vi "Staage 3.vi"() -> (0 "pass":bool=TRUE, 1 "Boolean 5":bool, 2 "Boolean 7":bool, 3 "Boolean 8":bool)   [LabVIEW 2014]
uses:
  <vilib>/Utility/miscctls.llb/LVPositionTypeDef.ctl
panel:
  in  "Position 2":T1={"Left"=24, "Top"=2148}
  in  "hh":dbl format="%0#2_6g"
  in  ":":dbl format="%0#2_6g"
  in  "ss":dbl format="%0#2_6g"
  in  "OK Button 112":bool
  out "Boolean 3":bool
  out "Boolean":bool
  out "Boolean 2":bool
  out "star 1":bool
  out "star 2":bool
  out "star 3":bool
  out "result":bool
  in  "Boolean 6":bool
  in  "Position":T1
  in  "Map Array":dbl[][](array[numeric])=array190x190[36100 elements]
  in  "OK Button 111":bool
  in  "OK Button 110":bool
  in  "OK Button 109":bool
  in  "OK Button 108":bool
  in  "OK Button 107":bool
  in  "OK Button 106":bool
  in  "OK Button 105":bool
  in  "OK Button 104":bool
  in  "OK Button 103":bool
  in  "OK Button 102":bool
  in  "OK Button 101":bool
  in  "OK Button 100":bool
  in  "OK Button 99":bool
  in  "OK Button 98":bool
  in  "OK Button 97":bool
  in  "OK Button 96":bool
  in  "OK Button 95":bool
  in  "OK Button 94":bool
  in  "stop 4":bool
  in  "OK Button 93":bool
  in  "OK Button 92":bool
  in  "OK Button 91":bool
  in  "OK Button 90":bool
  in  "OK Button 89":bool
  in  "OK Button 88":bool
  in  "OK Button 87":bool
  in  "OK Button 86":bool
  in  "OK Button 85":bool
  in  "OK Button 84":bool
  in  "OK Button 83":bool
  in  "OK Button 82":bool
  in  "OK Button 81":bool
  in  "OK Button 80":bool
  in  "OK Button 79":bool
  in  "OK Button 78":bool
  in  "OK Button 77":bool
  in  "OK Button 76":bool
  in  "OK Button 75":bool
  in  "OK Button 74":bool
  in  "OK Button 73":bool
  in  "stop 3":bool
  in  "stop 2":bool
  in  "OK Button 72":bool
  in  "OK Button 71":bool
  in  "OK Button 70":bool
  in  "OK Button 69":bool
  in  "OK Button 68":bool
  in  "OK Button 67":bool
  in  "OK Button 66":bool
  in  "OK Button 65":bool
  in  "OK Button 64":bool
  in  "OK Button 63":bool
  in  "OK Button 62":bool
  in  "OK Button 61":bool
  in  "OK Button 60":bool
  in  "OK Button 59":bool
  in  "OK Button 58":bool
  in  "OK Button 57":bool
  in  "OK Button 56":bool
  in  "OK Button 55":bool
  in  "OK Button 54":bool
  in  "OK Button 53":bool
  in  "OK Button 52":bool
  in  "OK Button 51":bool
  in  "OK Button 50":bool
  in  "OK Button 49":bool
  in  "OK Button 48":bool
  in  "OK Button 47":bool
  in  "OK Button 46":bool
  in  "OK Button 45":bool
  in  "OK Button 44":bool
  in  "OK Button 43":bool
  in  "OK Button 42":bool
  in  "OK Button 41":bool
  in  "OK Button 40":bool
  in  "OK Button 39":bool
  in  "OK Button 38":bool
  in  "OK Button 37":bool
  in  "OK Button 36":bool
  in  "OK Button 35":bool
  in  "OK Button 34":bool
  in  "OK Button 33":bool
  in  "OK Button 32":bool
  in  "OK Button 31":bool
  in  "OK Button 30":bool
  in  "OK Button 29":bool
  in  "OK Button 28":bool
  in  "OK Button 27":bool
  in  "OK Button 26":bool
  in  "OK Button 25":bool
  in  "OK Button 24":bool
  in  "OK Button 23":bool
  in  "OK Button 22":bool
  in  "OK Button 21":bool
  in  "OK Button 20":bool
  in  "OK Button 19":bool
  in  "OK Button 18":bool
  in  "OK Button 17":bool
  in  "OK Button 16":bool
  in  "OK Button 15":bool
  in  "OK Button 14":bool
  in  "OK Button 13":bool
  in  "OK Button 12":bool
  in  "OK Button 11":bool
  in  "OK Button 10":bool
  in  "OK Button 9":bool
  in  "OK Button 8":bool
  in  "OK Button 7":bool
  in  "OK Button 6":bool
  in  "OK Button 5":bool
  in  "OK Button 4":bool
  in  "OK Button 3":bool
  in  "OK Button 2":bool
  in  "character":bool
  in  "OK Button":bool
  out "Boolean 4":bool
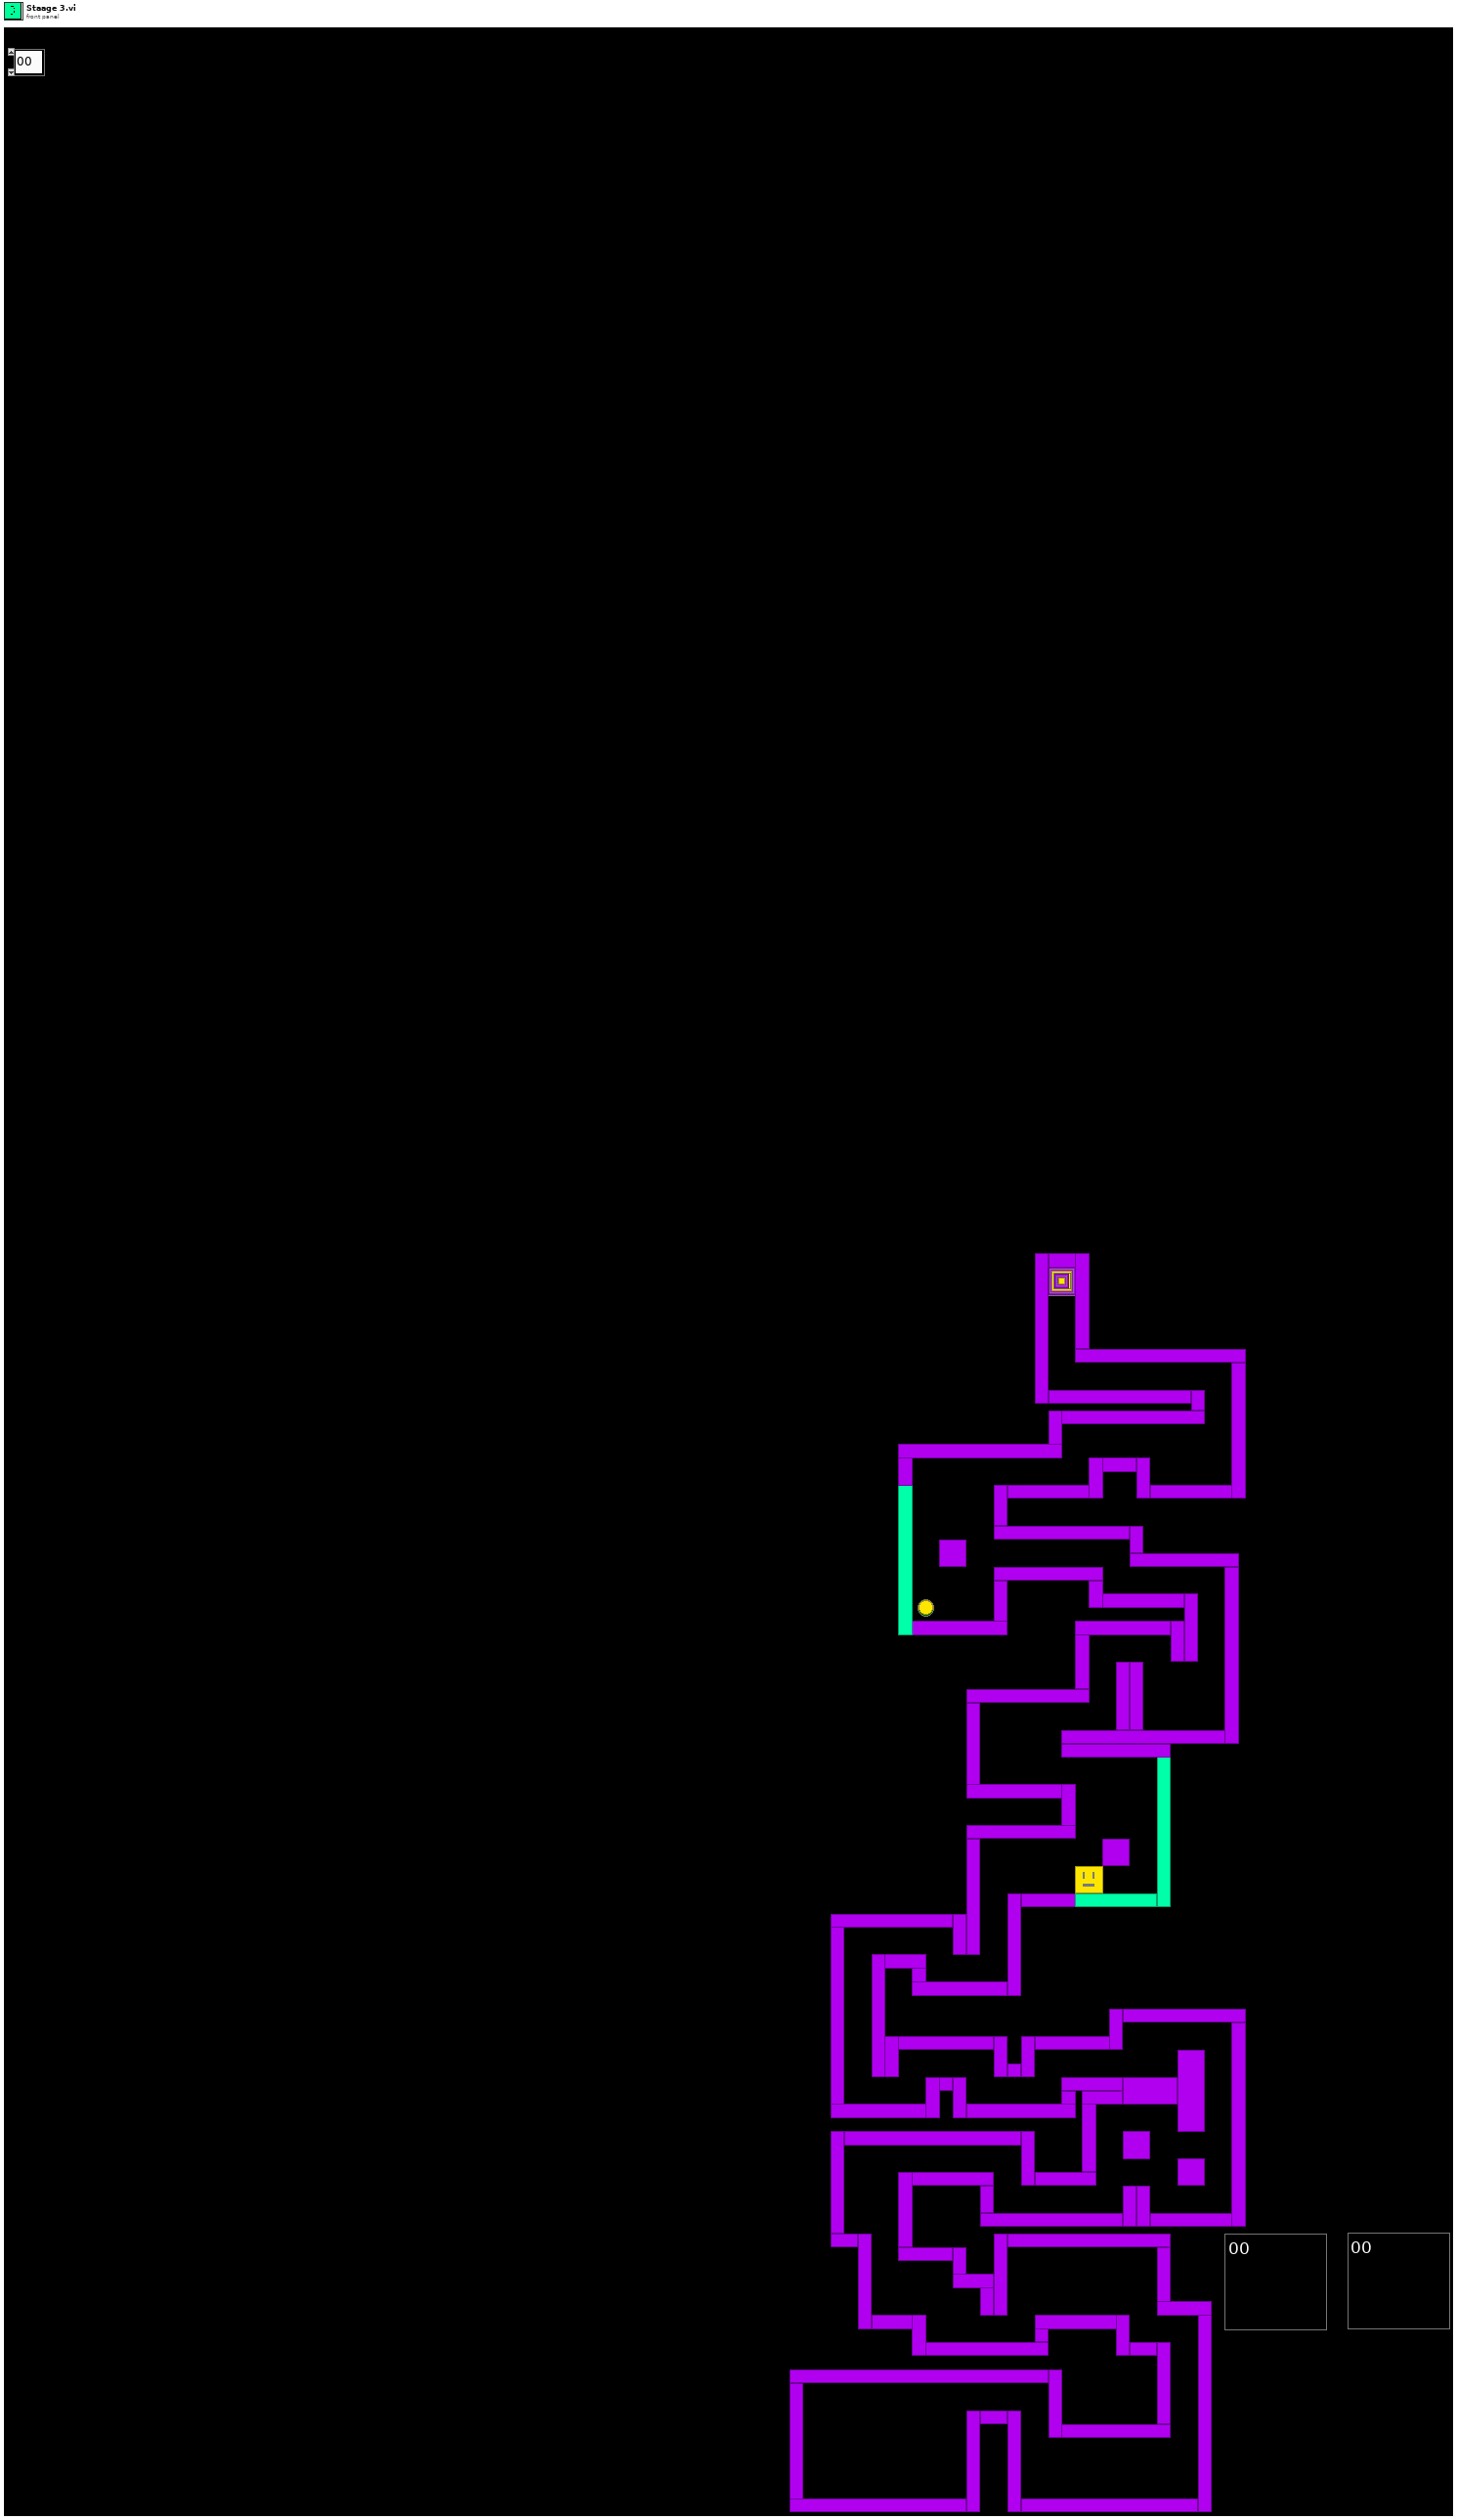
[diagram p1: front panel]
types:
  T1 = typedef "LVPositionTypeDef.ctl" = cluster{"Left":i32, "Top":i32}
  T2 = typedef "eventvkey.ctl" = enum16{"ASCII", "Enter", "Return", "Shift", "Ctrl", "Alt", "Cmd", "Opt", "Caps", "NumLock", "Clear", "Break", "Up", "Down", "Left", "Right", "Insert", "Delete", "Home", "End", "PageUp", "PageDown", "Escape", "Help", "Pause", "ScrollLock", "F1", "F2", "F3", "F4", "F5", "F6", "F7", "F8", "F9", "F10", "F11", "F12", "F13", "F14", "F15", "F16", "F17", "F18", "F19", "F20", "F21", "F22", "F23", "F24", "Play", "VolumeUp", "VolumeDown", "Mute", "Two Byte Char"}
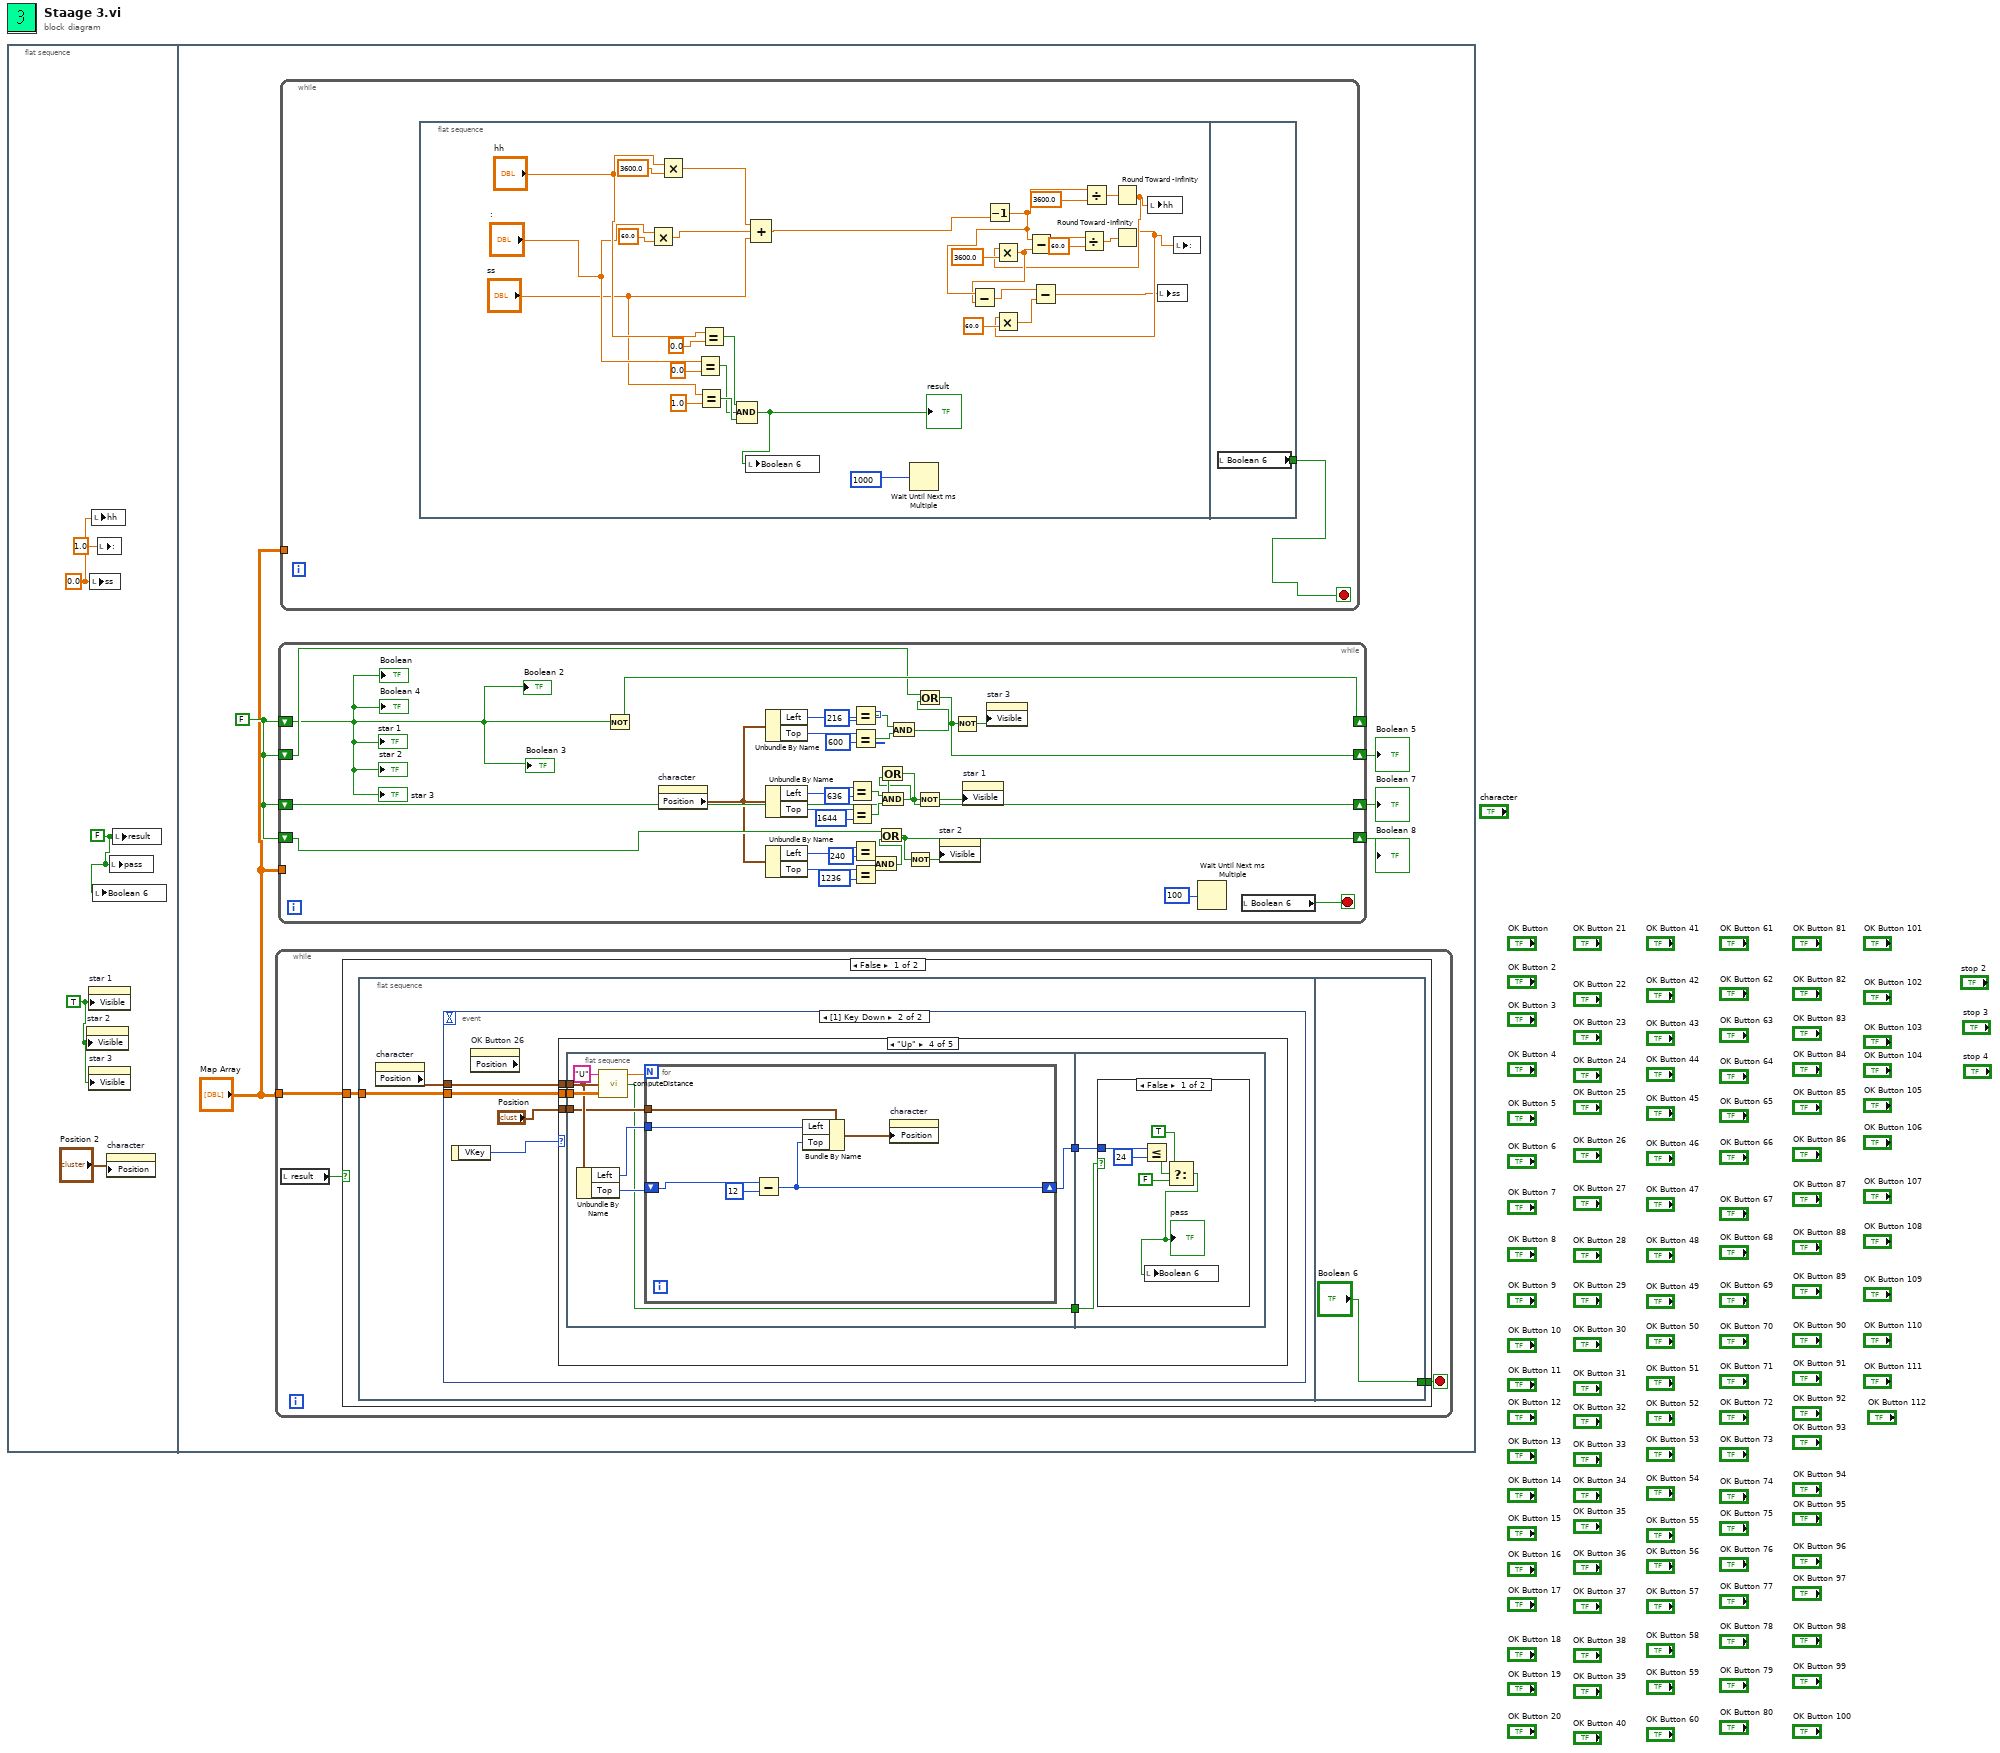
[diagram p0: block diagram]
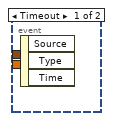
[diagram p2: hidden frame]
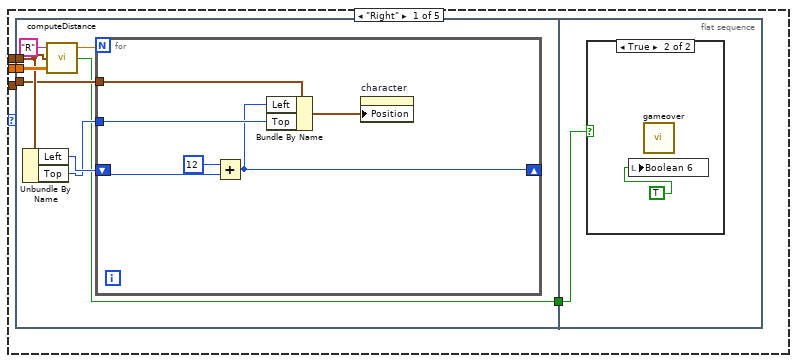
[diagram p3: hidden frame]
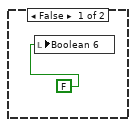
[diagram p4: hidden frame]
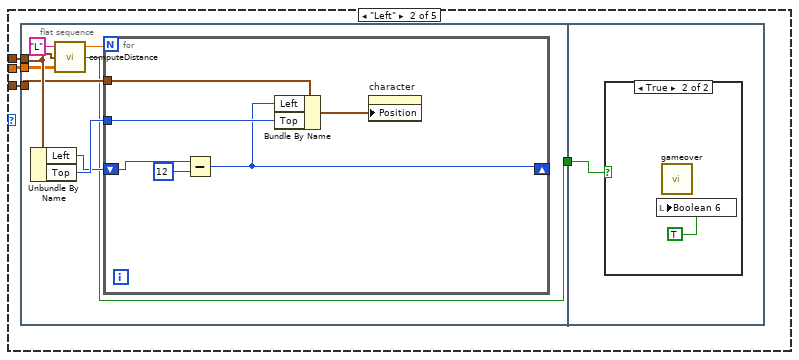
[diagram p5: hidden frame]
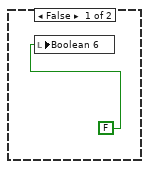
[diagram p6: hidden frame]
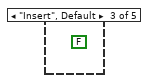
[diagram p7: hidden frame]
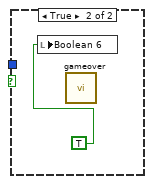
[diagram p8: hidden frame]
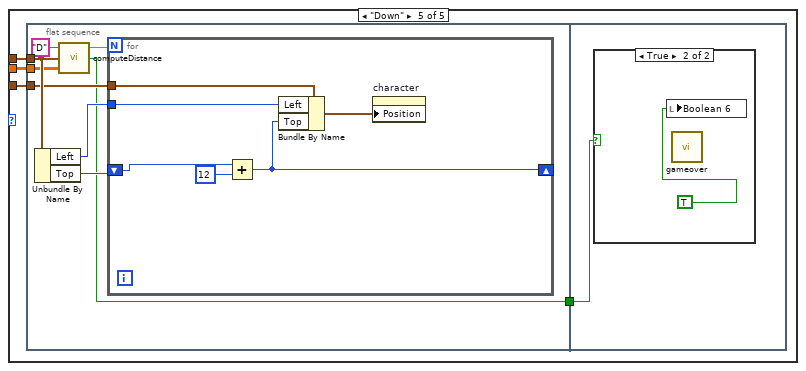
[diagram p9: hidden frame]
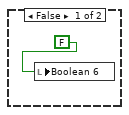
[diagram p10: hidden frame]
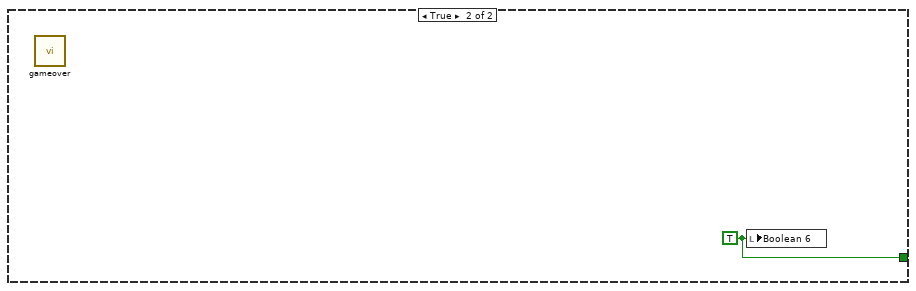
[diagram p11: hidden frame]
diagram:
  n1 = flat-sequence {
    frame #0 {
      w2 = TRUE ("Visible")
      w3 = FALSE ("result")
      w5 = 0.0 ("ss")
      n2 = property on="star 2" class="Bool (strict)"("Visible"=w2) -> ()  [unwired: 2 in, 2 out]
      n3 = property on="star 1" class="Bool (strict)"("Visible"=w2) -> ()  [unwired: 2 in, 2 out]
      n4 = property on="star 3" class="Bool (strict)"("Visible"=w2) -> ()  [unwired: 2 in, 2 out]
      n5 = local write "ss"(w5) -> ()
      n6 = local write "hh"(w5) -> ()
      n7 = local write "Boolean 6"(w3) -> ()
      n8 = local write ":"(1.0 (":")) -> ()
      n9 = property on="character" class="Bool"("Position"="Position 2") -> ()  [unwired: 2 in, 2 out]
      n10 = local write "pass"(w3) -> ()
      n11 = local write "result"(w3) -> ()
    }
    frame #1 {
      w10 = FALSE
      n12 = while {
        tunnel: "Map Array" -> [w80]
        stop <- w79 stop-if-true
        n13 = local read "result"() -> (w78:bool)
        n14 = case shown="False" w78 {
          tunnel: w80 -> [w82 _]
          tunnel: [w81 w182] -> w79
          frame False {
            n15 = flat-sequence {
              tunnel: w82 -> [w84]
              tunnel: ["Boolean 6"] -> w81
              frame #0 {
                n16 = property on="character" class="Bool"() -> ("Position"=w83:T1)  [unwired: 2 in, 2 out]
                n17 = event shown="[1] Key Down" {
                  selector: _ -> [_ _]
                  dyn-events: _ -> [_ _]
                  timeout: _ -> [_ _]
                  tunnel: w84 -> [_ w87]
                  tunnel: w83 -> [_ w86]
                  event Timeout {
                    n18 = event-data() -> ()  [unwired: 1 in, 3 out]
                  }
                  event Key Down {
                    n19 = event-data() -> ("VKey"=w88:T2)  [unwired: 1 in]
                    n20 = property on="OK Button 26" class="Bool" props=["Position"]() -> ()  [unwired: 2 in, 3 out]
                    n21 = case shown="\"Up\"" w88 {
                      tunnel: w87 -> [w92 w112 _ w135 w162]
                      tunnel: w86 -> [w91 w113 _ w134 w163]
                      tunnel: "Position" -> [w90 w111 _ w133 w161]
                      frame "Right" {
                        n22 = flat-sequence {
                          tunnel: w92 -> [w98]
                          tunnel: w91 -> [w97]
                          tunnel: w90 -> [w96]
                          tunnel: [w93] -> w89
                          tunnel: w89 -> [w107]
                          frame #0 {
                            n23 = Unbundle By Name(w97) -> ("Left"=w95:i32, "Top"=w94:i32)
                            n24 = call "computeDistance.vi"("Array"=w98, "Position"=w97, "String"="R") -> ("2"=w93:bool, "distance"=w100:dbl)  [unwired: 1 out]
                            n25 = for {
                              N: w100 -> [_]
                              shift-right: [w103] -> _
                              shift-left: w95 -> [w106]
                              tunnel: w96 -> [w105]
                              tunnel: w94 -> [w104]
                              n26 = Add(x=12, y=w106) -> (x+y=w103:i32)
                              n27 = Bundle By Name(cluster=w105, "Left"=w103, "Top"=w104) -> (w101:T1)
                              n28 = property on="character" class="Bool"("Position"=w101) -> ()  [unwired: 2 in, 2 out]
                            }
                          }
                          frame #1 {
                            n29 = case shown="True" w107 {
                              frame False {
                                n30 = local write "Boolean 6"(FALSE) -> ()
                              }
                              frame True {
                                n31 = local write "Boolean 6"(TRUE) -> ()
                                n32 = call "gameover.vi"() -> ()  [unwired: 1 in]
                              }
                            }
                          }
                        }
                      }
                      frame "Left" {
                        n33 = flat-sequence {
                          tunnel: w113 -> [w117]
                          tunnel: w112 -> [w116]
                          tunnel: w111 -> [w115]
                          tunnel: [w114] -> w110
                          tunnel: w110 -> [w128]
                          frame #0 {
                            n34 = Unbundle By Name(w117) -> ("Left"=w120:i32, "Top"=w121:i32)
                            n35 = call "computeDistance.vi"("Array"=w116, "Position"=w117, "String"="L") -> ("2"=w114:bool, "distance"=w118:dbl)  [unwired: 1 out]
                            n36 = for {
                              N: w118 -> [_]
                              shift-right: [w125] -> _
                              shift-left: w120 -> [w124]
                              tunnel: w115 -> [w127]
                              tunnel: w121 -> [w126]
                              n37 = Subtract(x=w124, y=12) -> (x-y=w125:i32)
                              n38 = Bundle By Name(cluster=w127, "Left"=w125, "Top"=w126) -> (w122:T1)
                              n39 = property on="character" class="Bool"("Position"=w122) -> ()  [unwired: 2 in, 2 out]
                            }
                          }
                          frame #1 {
                            n40 = case shown="True" w128 {
                              frame False {
                                n41 = local write "Boolean 6"(FALSE) -> ()
                              }
                              frame True {
                                n42 = local write "Boolean 6"(TRUE) -> ()
                                n43 = call "gameover.vi"() -> ()  [unwired: 1 in]
                              }
                            }
                          }
                        }
                      }
                      frame "Insert", Default {
                        (unwired) FALSE
                      }
                      frame "Up" {
                        n44 = flat-sequence {
                          tunnel: w135 -> [w144]
                          tunnel: w134 -> [w141]
                          tunnel: w133 -> [w138]
                          tunnel: [w137] -> w132
                          tunnel: [w136] -> w131
                          tunnel: w132 -> [w152]
                          tunnel: w131 -> [w151]
                          frame #0 {
                            n45 = Unbundle By Name(w141) -> ("Left"=w139:i32, "Top"=w140:i32)
                            n46 = call "computeDistance.vi"("Array"=w144, "Position"=w141, "String"="U") -> ("2"=w137:bool, "distance"=w142:dbl)  [unwired: 1 out]
                            n47 = for {
                              N: w142 -> [_]
                              shift-right: [w150] -> w136
                              shift-left: w140 -> [w147]
                              tunnel: w139 -> [w149]
                              tunnel: w138 -> [w148]
                              n48 = Subtract(x=w147, y=12) -> (x-y=w150:i32)
                              n49 = Bundle By Name(cluster=w148, "Left"=w149, "Top"=w150) -> (w145:T1)
                              n50 = property on="character" class="Bool"("Position"=w145) -> ()  [unwired: 2 in, 2 out]
                            }
                          }
                          frame #1 {
                            n51 = case shown="False" w152 {
                              tunnel: w151 -> [w158 _]
                              frame False {
                                n52 = Less Or Equal?(x=w158, y=24) -> (x <= y?=w156:bool)
                                n53 = Select(t=TRUE, s=w156, f=FALSE) -> (s? t:f=w154:bool)
                                "pass" <- w154
                                n54 = local write "Boolean 6"(w154) -> ()
                              }
                              frame True {
                                n55 = local write "Boolean 6"(TRUE) -> ()
                                n56 = call "gameover.vi"() -> ()  [unwired: 1 in]
                              }
                            }
                          }
                        }
                      }
                      frame "Down" {
                        n57 = flat-sequence {
                          tunnel: w163 -> [w167]
                          tunnel: w162 -> [w166]
                          tunnel: w161 -> [w165]
                          tunnel: [w164] -> w160
                          tunnel: w160 -> [w178]
                          frame #0 {
                            n58 = Unbundle By Name(w167) -> ("Left"=w171:i32, "Top"=w170:i32)
                            n59 = call "computeDistance.vi"("Array"=w166, "Position"=w167, "String"="D") -> ("2"=w164:bool, "distance"=w169:dbl)  [unwired: 1 out]
                            n60 = for {
                              N: w169 -> [_]
                              shift-right: [w177] -> _
                              shift-left: w170 -> [w174]
                              tunnel: w171 -> [w176]
                              tunnel: w165 -> [w175]
                              n61 = Add(x=w174, y=12) -> (x+y=w177:i32)
                              n62 = Bundle By Name(cluster=w175, "Left"=w176, "Top"=w177) -> (w172:T1)
                              n63 = property on="character" class="Bool"("Position"=w172) -> ()  [unwired: 2 in, 2 out]
                            }
                          }
                          frame #1 {
                            n64 = case shown="True" w178 {
                              frame False {
                                n65 = local write "Boolean 6"(FALSE ("Boolean 6")) -> ()
                              }
                              frame True {
                                n66 = local write "Boolean 6"(TRUE) -> ()
                                n67 = call "gameover.vi"() -> ()  [unwired: 1 in]
                              }
                            }
                          }
                        }
                      }
                    }
                  }
                }
              }
              frame #1 {
              }
            }
          }
          frame True {
            w182 = TRUE ("Boolean 6")
            n68 = call "gameover.vi"() -> ()  [unwired: 1 in]
            n69 = local write "Boolean 6"(w182) -> ()
          }
        }
      }
      n70 = while {
        shift-right: [w76] -> _
        shift-left: w10 -> [w43]
        shift-right: [w65] -> w8
        shift-left: w10 -> [w67]
        shift-right: [w56] -> w7
        shift-left: w10 -> [w55]
        shift-right: [w45] -> w9
        shift-left: w10 -> [w44]
        tunnel: "Map Array" -> [_]
        stop <- w75 stop-if-true
        n71 = Not(x=w43) -> (.not. x?=w76:bool)
        n72 = property on="character" class="Bool"() -> ("Position"=w46:T1)  [unwired: 2 in, 2 out]
        n73 = Unbundle By Name(w46) -> ("Left"=w54:i32, "Top"=w52:i32)
        n74 = Unbundle By Name(w46) -> ("Left"=w74:i32, "Top"=w72:i32)
        n75 = Unbundle By Name(w46) -> ("Left"=w57:i32, "Top"=w59:i32)
        n76 = Equal?(x=w74, y=636) -> (x = y?=w70:bool)
        n77 = Equal?(x=w72, y=1644) -> (x = y?=w69:bool)
        n78 = Equal?(x=w54, y=216) -> (x = y?=w50:bool)
        n79 = Equal?(x=w52, y=600) -> (x = y?=w49:bool)
        n80 = Equal?(x=w57, y=240) -> (x = y?=w61:bool)
        n81 = Equal?(x=w59, y=1236) -> (x = y?=w62:bool)
        n82 = And(x=w61, y=w62) -> (x .and. y?=w64:bool)
        n83 = Or(x=w55, y=w64) -> (x .or. y?=w56:bool)
        n84 = And(x=w70, y=w69) -> (x .and. y?=w66:bool)
        n85 = Or(x=w67, y=w66) -> (x .or. y?=w65:bool)
        n86 = And(x=w50, y=w49) -> (x .and. y?=w47:bool)
        n87 = Not(x=w56) -> (.not. x?=w63:bool)
        n88 = Not(x=w65) -> (.not. x?=w68:bool)
        n89 = Or(x=w44, y=w47) -> (x .or. y?=w45:bool)
        n90 = property on="star 2" class="Bool (strict)"("Visible"=w63) -> ()  [unwired: 2 in, 2 out]
        n91 = Not(x=w45) -> (.not. x?=w48:bool)
        n92 = property on="star 1" class="Bool (strict)"("Visible"=w68) -> ()  [unwired: 2 in, 2 out]
        n93 = property on="star 3" class="Bool (strict)"("Visible"=w48) -> ()  [unwired: 2 in, 2 out]
        n94 = Wait Until Next ms Multiple(millisecond multiple=u32 100) -> ()  [unwired: 1 out]
        n95 = local read "Boolean 6"() -> (w75:bool)
        "star 1" <- w43
        "star 2" <- w43
        "star 3" <- w43
        "Boolean" <- w43
        "Boolean 4" <- w43
        "Boolean 2" <- w43
        "Boolean 3" <- w43
      }
      "Boolean 5" <- w9
      "Boolean 7" <- w8
      "Boolean 8" <- w7
      n96 = while {
        tunnel: "Map Array" -> [_]
        stop <- w11 stop-if-true
        n97 = flat-sequence {
          tunnel: [w42] -> w11
          frame #0 {
            n98 = Multiply(x=":", y=60.0) -> (x*y=w40:dbl)
            n99 = Multiply(x="hh", y=3600.0) -> (x*y=w41:dbl)
            n100 = Equal?(x=":", y=0.0) -> (x = y?=w32:bool)
            n101 = Equal?(x="ss", y=1.0) -> (x = y?=w33:bool)
            n102 = Equal?(x="hh", y=0.0) -> (x = y?=w31:bool)
            n103 = Compound Arithmetic op=AND(w31, w32, w33) -> (w12:bool)
            "result" <- w12
            n104 = local write "Boolean 6"(w12) -> ()
            n105 = Compound Arithmetic op=ADD(w41, w40, "ss") -> (w37:dbl)
            n106 = Wait Until Next ms Multiple(millisecond multiple=u32 1000) -> ()  [unwired: 1 out]
            n107 = Decrement(x=w37) -> (x-1=w26:dbl)
            n108 = Divide(x=w26, y=3600.0) -> (x/y=w16:dbl)
            n109 = Round Toward -Infinity(1:w16) -> (0:w15:dbl)
            n110 = Multiply(x=w15, y=3600.0) -> (x*y=w22:dbl)
            n111 = Subtract(x=w26, y=w22) -> (x-y=w23:dbl)
            n112 = Subtract(x=w26, y=w22) -> (x-y=w19:dbl)
            n113 = Divide(x=w19, y=60.0) -> (x/y=w21:dbl)
            n114 = Round Toward -Infinity(1:w21) -> (0:w14:dbl)
            n115 = Multiply(x=w14, y=60.0) -> (x*y=w25:dbl)
            n116 = Subtract(x=w23, y=w25) -> (x-y=w13:dbl)
            n117 = local write "hh"(w15) -> ()
            n118 = local write "ss"(w13) -> ()
            n119 = local write ":"(w14) -> ()
          }
          frame #1 {
            n120 = local read "Boolean 6"() -> (w42:bool)
          }
        }
      }
    }
  }
